vi "Scanner Box(1ST) Test for MANU.vi"(8 "error in":errorcluster, 11 "VISA resource name":refnum<visa-resource-name>) -> (0 "error out":errorcluster, 3 "VISA resource name out":refnum<visa-resource-name>)   [LabVIEW 2011, in "GPT-9000.lvlib"]
uses:
  <instrlib>/GPT-9000/GPT-9000.lvlib
panel:
  out "Model Type of 1ST":string
  out "Error Message":string
  out "CH8_1_F":bool caption="Fail"
  out "CH8_1_P":bool caption="CH8"
  out "CH7_1_F":bool caption="Fail"
  out "CH7_1_P":bool caption="CH7"
  out "CH6_1_F":bool caption="Fail"
  out "CH6_1_P":bool caption="CH6"
  out "CH5_1_F":bool caption="Fail"
  out "CH5_1_P":bool caption="CH5"
  out "CH4_1_F":bool caption="Fail"
  out "CH4_1_P":bool caption="CH4"
  out "CH3_1_F":bool caption="Fail"
  out "CH3_1_P":bool caption="CH3"
  out "CH2_1_F":bool caption="Fail"
  out "CH2_1_P":bool caption="CH2"
  out "CH1_1_F":bool caption="Fail"
  out "CH1_1_P":bool caption="CH1"
  out "read buffer":string
  in  "Test number":u8=1 max=100
  out "ID Return String":string
  in  "Configure RS232 Baud Rate":u32(ring)=115200 items=["9600"=9600, "19200"=19200, "38400"=38400, "57600"=57600, "115200"=115200]
  in  "Clear Error(True)":bool=TRUE
  in  "ID Query (True)":bool=TRUE
  # "PASS"
  # "BOX(1ST)"
  # "FAIL"
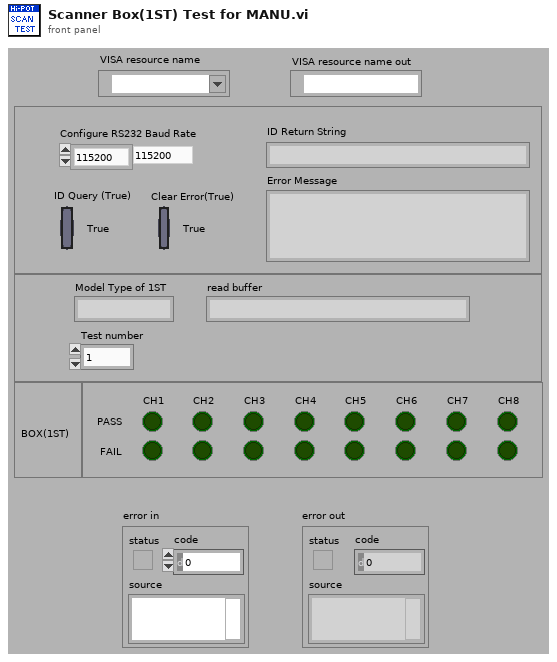
[diagram p1: front panel]
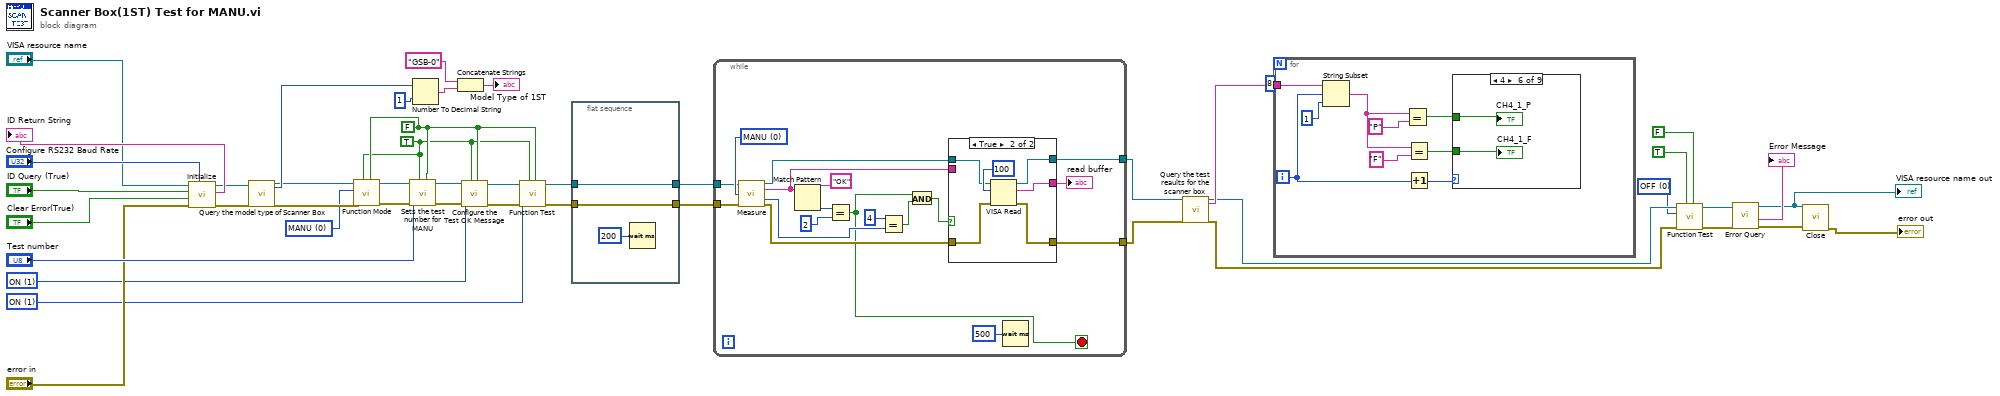
[diagram p0: block diagram]
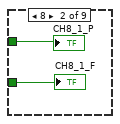
[diagram p3: hidden frame]
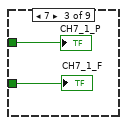
[diagram p4: hidden frame]
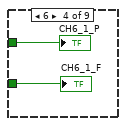
[diagram p5: hidden frame]
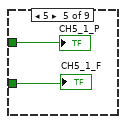
[diagram p6: hidden frame]
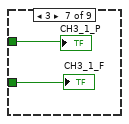
[diagram p7: hidden frame]
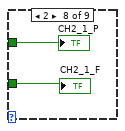
[diagram p8: hidden frame]
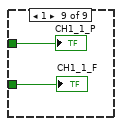
[diagram p9: hidden frame]
diagram:
  w3 = u8 0 items=["AUTO"=1, "MANU"=0] ("Function Mode")
  w15 = u8 0 items=["OFF", "ON"] ("Function Test")
  w34 = u8 1 items=["OFF", "ON"] ("Function Test")
  w39 = u8 1 items=["OFF", "ON"] ("Send Message when test stop")
  w2 = FALSE
  w1 = TRUE
  n1 = call <instrlib>:"Initialize.vi"("Configure RS232 Baud Rate"="Configure RS232 Baud Rate", "error in (no error)"="error in", "Clear Error(True)"="Clear Error(True)", "ID Query (True)"="ID Query (True)", "VISA resource name"="VISA resource name") -> ("error out"=w27:errorcluster, "ID Return String"=→"ID Return String":string, "VISA resource name out"=w28:refnum<visa-resource-name>)  [unwired: 3 in, 1 out]
  n2 = call <instrlib>:"Query the model type of Scanner Box.vi"("VISA resource name"=w28, "error in"=w27) -> ("VISA resource name out"=w7:refnum<visa-resource-name>, "Model Type of 1ST"=w26:i32, "error out"=w6:errorcluster)  [unwired: 12 in, 3 out]
  n3 = call <instrlib>:"Function Mode.vi"("Enable to Query"=w2, "Enable to Setup"=w1, "error in"=w6, "Function Mode"=w3, "VISA resource name"=w7) -> ("error out"=w4:errorcluster, "VISA resource name out"=w5:refnum<visa-resource-name>)  [unwired: 4 in, 1 out]
  n4 = call <instrlib>:"Sets the test number for MANU.vi"("Enable to Query"=w2, "Enable to Setup"=w1, "error in"=w4, "Test number"="Test number", "VISA resource name"=w5) -> ("error out"=w37:errorcluster, "VISA resource name out"=w38:refnum<visa-resource-name>)  [unwired: 4 in, 1 out]
  n5 = Number To Decimal String(number=w26, width (-)=i16 1) -> (decimal integer string=w23:string)
  n6 = Concatenate Strings("GSB-0" ("string"), w23) -> (→"Model Type of 1ST":string)
  n7 = call <instrlib>:"Configure the Test OK Message.vi"("Query the Message"=w2, "Setup the Message"=w1, "error in"=w37, "Send Message when test stop"=w39, "VISA resource name"=w38) -> ("error out"=w35:errorcluster, "VISA resource name out"=w36:refnum<visa-resource-name>)  [unwired: 4 in, 1 out]
  n8 = call <instrlib>:"Function Test.vi"("VISA resource name"=w36, "Function Test"=w34, "error in"=w35, "Enable to Setup"=w1, "Enable to Query"=w2) -> ("VISA resource name out"=w21:refnum<visa-resource-name>, "error out"=w20:errorcluster)  [unwired: 3 in, 1 out]
  n9 = flat-sequence {
    tunnel: w21 -> [w48]
    tunnel: w20 -> [w47]
    tunnel: [w48] -> w19
    tunnel: [w47] -> w18
    frame #0 {
      n10 = Wait (ms)(milliseconds to wait=u32 200) -> ()  [unwired: 1 out]
    }
  }
  n11 = while {
    tunnel: w19 -> [w56]
    tunnel: w18 -> [w55]
    tunnel: [w54] -> w33
    tunnel: [w53] -> w32
    stop <- w51 stop-if-true
    w67 = u8 0 items=["MANU", "AUTO"] ("Function Mode Numeric")
    n12 = call <instrlib>:"Measure.vi"("VISA resource name"=w56, "Function Mode Numeric"=w67, "error in"=w55) -> ("VISA resource name out"=w63:refnum<visa-resource-name>, "Return  the test status"=w57:string, "Return the String Count"=w59:u16, "error out"=w62:errorcluster)  [unwired: 9 in]
    n13 = Match Pattern(string=w57, regular expression="OK") -> (offset past match=w65:i32)  [unwired: 1 in, 3 out]
    n14 = Equal?(x=w65, y=2) -> (x = y?=w51:bool)
    n15 = Equal?(x=u16 4, y=w59) -> (x = y?=w60:bool)
    n16 = And(x=w51, y=w60) -> (x .and. y?=w61:bool)
    n17 = case shown="True" w61 {
      tunnel: w62 -> [w70 w71]
      tunnel: [w69 w75] -> w54
      tunnel: [w70 w74] -> w53
      tunnel: [w68 w73] -> w50
      tunnel: w63 -> [w69 w72]
      tunnel: w57 -> [w68 _]
      frame False {
      }
      frame True {
        n18 = VISA Read(VISA resource name=w72, byte count=u32 100, error in (no error)=w71) -> (VISA resource name out=w75:refnum<visa-resource-name>, read buffer=w73:string, error out=w74:errorcluster)  [unwired: 1 out]
      }
    }
    "read buffer" <- w50
    n19 = Wait (ms)(milliseconds to wait=u32 500) -> ()  [unwired: 1 out]
  }
  n20 = call <instrlib>:"Query the test reaults for the scanner box.vi"("VISA resource name"=w33, "error in"=w32) -> ("VISA resource name out"=w17:refnum<visa-resource-name>, "Test Results for 1ST"=w30:string, "error out"=w16:errorcluster)  [unwired: 12 in, 3 out]
  n21 = for {
    N: 8 -> [_]
    tunnel: w30 -> [w85]
    i -> [w80]
    n22 = String Subset(string=w85, offset (0)=w80, length (rest)=1 ("length (rest)")) -> (substring=w83:string)
    n23 = Equal?(x=w83, y="P") -> (x = y?=w78:bool)
    n24 = Equal?(x=w83, y="F") -> (x = y?=w77:bool)
    n25 = Increment(x=w80) -> (x+1=w79:i32)
    n26 = case shown="4" w79 {
      tunnel: w78 -> [_ w87 w89 w91 w93 w95 w97 w99 w101]
      tunnel: w77 -> [_ w86 w88 w90 w92 w94 w96 w98 w100]
      frame 0, Default {
      }
      frame 8 {
        "CH8_1_P" <- w87
        "CH8_1_F" <- w86
      }
      frame 7 {
        "CH7_1_P" <- w89
        "CH7_1_F" <- w88
      }
      frame 6 {
        "CH6_1_P" <- w91
        "CH6_1_F" <- w90
      }
      frame 5 {
        "CH5_1_P" <- w93
        "CH5_1_F" <- w92
      }
      frame 4 {
        "CH4_1_P" <- w95
        "CH4_1_F" <- w94
      }
      frame 3 {
        "CH3_1_P" <- w97
        "CH3_1_F" <- w96
      }
      frame 2 {
        "CH2_1_P" <- w99
        "CH2_1_F" <- w98
      }
      frame 1 {
        "CH1_1_P" <- w101
        "CH1_1_F" <- w100
      }
    }
  }
  n27 = call <instrlib>:"Function Test.vi"("VISA resource name"=w17, "Function Test"=w15, "error in"=w16, "Enable to Setup"=TRUE, "Enable to Query"=FALSE) -> ("VISA resource name out"=w12:refnum<visa-resource-name>, "error out"=w11:errorcluster)  [unwired: 3 in, 1 out]
  n28 = call <instrlib>:"Error Query.vi"("error in (no error)"=w11, "VISA resource name"=w12) -> ("error out"=w10:errorcluster, "Error Message"=→"Error Message":string, "VISA resource name out"=w8:refnum<visa-resource-name>)  [unwired: 6 in, 1 out]
  "VISA resource name out" <- w8
  n29 = call <instrlib>:"Close.vi"("error in (no error)"=w10, "VISA resource name"=w8) -> ("error out"=→"error out":errorcluster)  [unwired: 9 in]
